vi "MatchEnumIndexToString.vi"(10 "Enum Variant":variant, 11 "String":string) -> (2 "found":bool, 3 "index":i32)   [LabVIEW 2020, in "openg_variant.lvlib"]
uses:
  openg_variant.lvlib
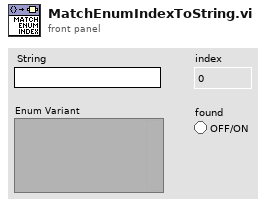
[diagram p1: front panel]
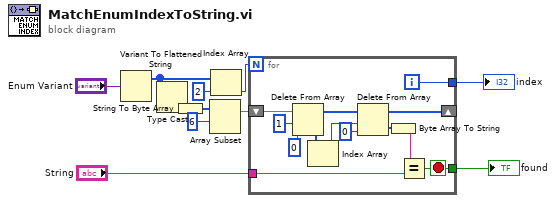
[diagram p0: block diagram]
diagram:
  n1 = Variant To Flattened String(Variant="Enum Variant") -> (1:w4:i16[])  [unwired: 1 out]
  n2 = Type Cast(x=w4) -> (*(type *) &x=w8:string)  [unwired: 1 in]
  n3 = String To Byte Array(string=w8) -> (unsigned byte array=w7:u8[])
  n4 = Array Subset(array=w7, index=6) -> (w6:u8[])  [unwired: 1 in]
  n5 = Index Array(array=w4, index=2) -> (element=w9:i16)
  n6 = for {
    N: w9 -> [_]
    shift-right: [w18] -> _
    shift-left: w6 -> [w24]
    tunnel: "String" -> [w14]
    tunnel: [w13] -> w10
    tunnel: [w12] -> w11
    i -> [w13]
    stop <- w12 stop-if-true
    n7 = Delete From Array(array=w24, length=1, index=0) -> (deleted portion=w21:u8[], array with subset deleted=w20:u8[])
    n8 = Index Array(array=w21) -> (element=w19:u8)  [unwired: 1 in]
    n9 = Delete From Array(array=w20, length=w19, index=0) -> (deleted portion=w16:u8[], array with subset deleted=w18:u8[])
    n10 = Byte Array To String(unsigned byte array=w16) -> (string=w15:string)
    n11 = Equal?(x=w15, y=w14) -> (x = y?=w12:bool)
  }
  "found" <- w11
  "index" <- w10
